vi "Run.vi"(8 "error in (no error)":errorcluster, 10 "TestResult":refnum<class "TestResult.lvclass">, 11 "Test In":refnum<class "Test.lvclass">) -> (0 "error out":errorcluster, 2 "TestResult out":refnum<class "TestResult.lvclass">, 3 "Test Out":refnum<class "Test.lvclass">)   [LabVIEW 2019, in "Test.lvclass"]
doc: "Runs the test and collects results in a <B>TestResult</B> object."
uses:
  Test.lvclass
  TestResult/TestResult.lvclass
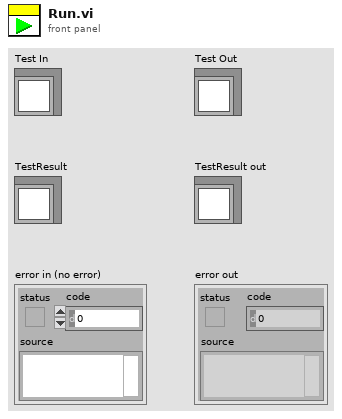
[diagram p1: front panel]
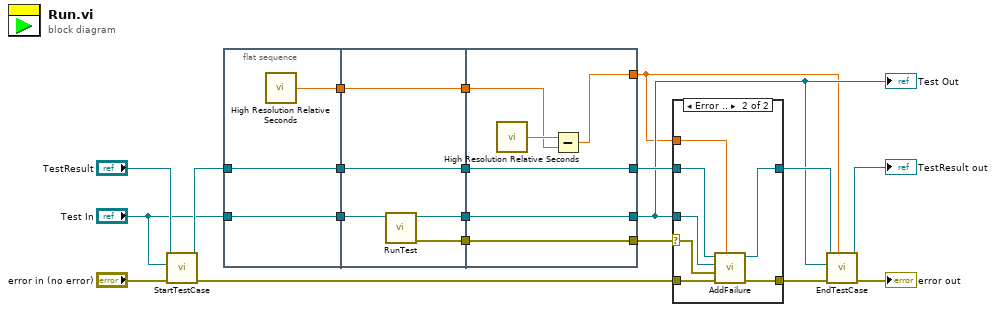
[diagram p0: block diagram]
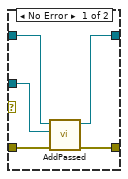
[diagram p2: hidden frame]
diagram:
  n1 = call-dynamic "StartTestCase.vi"("error in (no error)"="error in (no error)", "Test"="Test In", "TestResult in"="TestResult") -> ("error out"=w10:errorcluster, "TestResult out"=w8:refnum<class "TestResult.lvclass">)  [unwired: 7 in]
  n2 = flat-sequence {
    tunnel: w8 -> [w22]
    tunnel: "Test In" -> [w23]
    tunnel: [w23] -> w20
    tunnel: [w22] -> w19
    tunnel: [w21] -> w18
    tunnel: [w27] -> w17
    tunnel: [w26] -> w16
    tunnel: [w24] -> w15
    tunnel: [w25] -> w14
    tunnel: w20 -> [w28]
    tunnel: w19 -> [w25]
    tunnel: w18 -> [w24]
    tunnel: [w34] -> w13
    tunnel: [w31] -> w2
    tunnel: w17 -> [w31]
    tunnel: w16 -> [w34]
    tunnel: w15 -> [w32]
    tunnel: w14 -> [w30]
    tunnel: [w30] -> w12
    tunnel: [w29] -> w1
    frame #0 {
      n3 = call <vilib>:"High Resolution Relative Seconds.vi"() -> ("relative seconds"=w21:dbl)
    }
    frame #1 {
      n4 = call-dynamic "RunTest.vi"("Test In"=w28) -> ("error out"=w26:errorcluster, "Test Out"=w27:refnum<class "Test.lvclass">)  [unwired: 9 in]
    }
    frame #2 {
      n5 = call <vilib>:"High Resolution Relative Seconds.vi"() -> ("relative seconds"=w33:dbl)
      n6 = Subtract(x=w33, y=w32) -> (x-y=w29:dbl)
    }
  }
  n7 = case shown="Error .." w13 {
    selector: w13 -> [_ w46]
    tunnel: [w36 w42] -> w4
    tunnel: w12 -> [w37 w43]
    tunnel: w10 -> [w39 w45]
    tunnel: w2 -> [w35 w44]
    tunnel: [w38 w41] -> w6
    tunnel: w1 -> [_ w40]
    frame No Error {
      n8 = call-dynamic "AddPassed.vi"("error in (no error)"=w39, "Test"=w35, "TestResult in"=w37) -> ("error out"=w38:errorcluster, "TestResult out"=w36:refnum<class "TestResult.lvclass">)  [unwired: 7 in]
    }
    frame Error {
      n9 = call-dynamic "AddFailure.vi"("Time"=w40, "error in (no error)"=w45, "Failure"=w46, "Test"=w44, "TestResult in"=w43) -> ("error out"=w41:errorcluster, "TestResult out"=w42:refnum<class "TestResult.lvclass">)  [unwired: 5 in]
    }
  }
  n10 = call-dynamic "EndTestCase.vi"("Time"=w1, "error in (no error)"=w6, "Test"=w2, "TestResult in"=w4) -> ("error out"=→"error out":errorcluster, "TestResult out"=→"TestResult out":refnum<class "TestResult.lvclass">)  [unwired: 6 in]
  "Test Out" <- w2
